vi "Initialize CAN Parameters.vi"(8 "error in (no error)":errorcluster, 11 "Diagnostics Basic Configuraiton":T24) -> (0 "error out":errorcluster, 3 "Configuration":T1={"Name"="", "Description"="", "Diagnostics Basic Configuraiton"={"Database File"=path "", "CAN Interface"=enum."CAN0", "Baud Rate"=0, "Diagnostic Protocol"=enum."GMLAN", "Transport Protocol"=enum."ISO TP - Normal Mode", "Transmit ID"=0, "Receive ID"=0, "Transmit Extension"=0, "Receive Extension"=0, "Receive UUDT ID"=0, "Enable Stream"=TRUE, "VW TP Channel ID"=0, "Security"={"DLL Path"=path "", "Security Level"=1}}, "DIDs"={"Description"="", "Frames"=[]}, "Input PIDs"={"Description"="", "Frames"=[]}, "Output PIDs"={"Description"="", "Frames"=[]}, "DPIDs"={"Description"="", "DPIDs"=[]}, "DTC"={"Description"="", "DTC descriptor"={"DTC Byte Length"=2, "Status Byte Length"=1, "Add Data Byte Length"=1, "Byte Order"=enum."Motorola"}}, "NI 986x Support"={"Enable 986x"=FALSE, "RIO Device"=0, "Bitfile"=path ""}, "Commands"={"Description"=""}, "Status"={"Description"=""}, "IO Controls"={"Description"="", "IO Control Array"=[]}, "Routines"={"Description"="", "Routine Array"=[]}, "Output Memory"={"Description"="", "Frames"=[]}, "Input Memory"={"Description"="", "Frames"=[]}} {"Input Memory"."Frames"."Signals"."Byte Order" items=["Little Endian", "Big Endian"]; "Input Memory"."Frames"."Signals"."Data Type" items=["Signed", "Unsigned", "IEEE Float"]; "Output Memory"."Frames"."Signals"."Byte Order" items=["Little Endian", "Big Endian"]; "Output Memory"."Frames"."Signals"."Data Type" items=["Signed", "Unsigned", "IEEE Float"]; "Routines"."Routine Array"."Stop Parameters"."Response"."Byte Order" items=["Little Endian", "Big Endian"]; "Routines"."Routine Array"."Stop Parameters"."Response"."Data Type" items=["Signed", "Unsigned", "IEEE Float"]; "Routines"."Routine Array"."Stop Parameters"."Cmd"."Byte Order" items=["Little Endian", "Big Endian"]; "Routines"."Routine Array"."Stop Parameters"."Cmd"."Data Type" items=["Signed", "Unsigned", "IEEE Float"]; "Routines"."Routine Array"."Request Parameters"."Response"."Byte Order" items=["Little Endian", "Big Endian"]; "Routines"."Routine Array"."Request Parameters"."Response"."Data Type" items=["Signed", "Unsigned", "IEEE Float"]; "Routines"."Routine Array"."Request Parameters"."Cmd"."Byte Order" items=["Little Endian", "Big Endian"]; "Routines"."Routine Array"."Request Parameters"."Cmd"."Data Type" items=["Signed", "Unsigned", "IEEE Float"]; "Routines"."Routine Array"."Start Parameters"."Response"."Byte Order" items=["Little Endian", "Big Endian"]; "Routines"."Routine Array"."Start Parameters"."Response"."Data Type" items=["Signed", "Unsigned", "IEEE Float"]; "Routines"."Routine Array"."Start Parameters"."Cmd"."Byte Order" items=["Little Endian", "Big Endian"]; "Routines"."Routine Array"."Start Parameters"."Cmd"."Data Type" items=["Signed", "Unsigned", "IEEE Float"]; "IO Controls"."IO Control Array"."Signals"."Response"."Byte Order" items=["Little Endian", "Big Endian"]; "IO Controls"."IO Control Array"."Signals"."Response"."Data Type" items=["Signed", "Unsigned", "IEEE Float"]; "IO Controls"."IO Control Array"."Signals"."Cmd"."Byte Order" items=["Little Endian", "Big Endian"]; "IO Controls"."IO Control Array"."Signals"."Cmd"."Data Type" items=["Signed", "Unsigned", "IEEE Float"]; "Diagnostics Basic Configuraiton"."VW TP Channel ID" format="%.0x"; "Diagnostics Basic Configuraiton"."Receive UUDT ID" format="%.0x"; "Diagnostics Basic Configuraiton"."Receive Extension" format="%.0x"; "Diagnostics Basic Configuraiton"."Transmit Extension" format="%.0x"; "Diagnostics Basic Configuraiton"."Receive ID" format="%.0x"; "Diagnostics Basic Configuraiton"."Transmit ID" format="%.0x"; "DIDs"."Frames"."Signals"."Byte Order" items=["Little Endian", "Big Endian"]; "DIDs"."Frames"."Signals"."Data Type" items=["Signed", "Unsigned", "IEEE Float"]; "Input PIDs"."Frames"."Signals"."Byte Order" items=["Little Endian", "Big Endian"]; "Input PIDs"."Frames"."Signals"."Data Type" items=["Signed", "Unsigned", "IEEE Float"]; "Output PIDs"."Frames"."Signals"."Byte Order" items=["Little Endian", "Big Endian"]; "Output PIDs"."Frames"."Signals"."Data Type" items=["Signed", "Unsigned", "IEEE Float"]})   [LabVIEW 2015, in "Diagnostics Addon System Explorer.lvlib"]
uses:
  Diagnostics Addon System Explorer.lvlib
  Shared/Base Configuration.ctl
  Shared/CAN Interface.ctl
  Shared/Diagnostic Protocols.ctl
  Shared/Exported Configuration.ctl
  Shared/CAN Configuration.ctl
  Shared/Transport Protocols.ctl
  Shared/Security.ctl
  Shared/Exported Frames Cluster.ctl
  Shared/Frame Parameters.ctl
  Shared/Signal Parameters.ctl
  Shared/Exported DPIDs Cluster.ctl
  Shared/Exported DPID Parameters.ctl
  Shared/DPID Parameters.ctl
  Shared/DPID Periodic Rate.ctl
  Shared/Exported DTC Cluster.ctl
  <vilib>/Automotive Diagnostic Command Set/Diagnostic Protocols.llb/DTC Descriptor.ctl
  Shared/Exported 986x Support.ctl
  Shared/Exported Command Cluster.ctl
  Shared/Exported Status Cluster.ctl
  Shared/Exported IO Control Cluster.ctl
  Shared/IO Control Parameters.ctl
  Shared/Input and Output Signal Parameters.ctl
  Shared/Exported Routines Cluster.ctl
  Shared/Routine Paramaters.ctl
  Shared/Diagnostics Addon Shared.lvlib
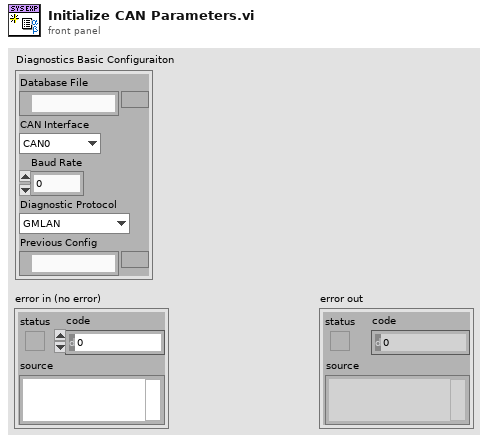
[diagram p1: front panel]
types:
  T1 = typedef "Diagnostics Addon System Explorer.lvlib/Exported Configuration.ctl" = cluster{"Name":string, "Description":string, "Diagnostics Basic Configuraiton":T2, "DIDs":T7, "Input PIDs":T7, "Output PIDs":T7, "DPIDs":T10, "DTC":T14, "NI 986x Support":T16, "Commands":T17, "Status":T18, "IO Controls":T19, "Routines":T22, "Output Memory":T7, "Input Memory":T7}
  T2 = typedef "Diagnostics Addon Shared.lvlib/CAN Configuration.ctl" = cluster{"Database File":path, "CAN Interface":T3, "Baud Rate":u32, "Diagnostic Protocol":T4, "Transport Protocol":T5, "Transmit ID":u32, "Receive ID":u32, "Transmit Extension":u8, "Receive Extension":u8, "Receive UUDT ID":u32, "Enable Stream":bool, "VW TP Channel ID":u32, "Security":T6}
  T3 = typedef "Diagnostics Addon Shared.lvlib/CAN Interface.ctl" = enum16{"CAN0", "CAN1", "CAN2", "CAN3", "CAN4", "CAN5", "CAN6", "CAN7", "CAN8", "CAN9", "CAN10", "CAN11", "CAN12", "CAN13", "CAN14", "CAN15", "CAN16", "CAN17", "CAN18", "CAN19", "CAN20", "CAN21", "CAN22", "CAN23", "CAN24", "CAN25", "CAN26", "CAN27", "CAN28", "CAN29", "CAN30", "CAN31", "CAN32", "CAN33", "CAN34", "CAN35", "CAN36", "CAN37", "CAN38", "CAN39", "CAN40", "CAN41", "CAN42", "CAN43", "CAN44", "CAN45", "CAN46", "CAN47", "CAN48", "CAN49", "CAN50", "CAN51", "CAN52", "CAN53", "CAN54", "CAN55", "CAN56", "CAN57", "CAN58", "CAN59", "CAN60", "CAN61", "CAN62", "CAN63", "CAN 256 (Virtual)", "CAN 257 (Virtual)"}
  T4 = typedef "Diagnostics Addon Shared.lvlib/Diagnostic Protocols.ctl" = enum16{"GMLAN", "KWP-2000", "UDS"}
  T5 = typedef "Diagnostics Addon Shared.lvlib/Transport Protocols.ctl" = enum16{"ISO TP - Normal Mode", "ISO TP - Mixed Mode", "VW TP 2.0", "Diagnostics on IP"}
  T6 = typedef "Diagnostics Addon Shared.lvlib/Security.ctl" = cluster{"DLL Path":path, "Security Level":u8}
  T7 = typedef "Diagnostics Addon System Explorer.lvlib/Exported Frames Cluster.ctl" = cluster{"Description":string, "Frames":T8[]}
  T8 = typedef "Diagnostics Addon Shared.lvlib/Frame Parameters.ctl" = cluster{"Name":string, "Description":string, "ID":u16, "Signals":T9[]}
  T9 = typedef "Diagnostics Addon Shared.lvlib/Signal Parameters.ctl" = cluster{"Start Bit":u8, "Length":u8, "Scaling Factor":dbl, "Scaling Offset":dbl, "Minimum":dbl, "Maximum":dbl, "Data Type":u32, "Byte Order":u32, "Default Value":dbl, "Name":string, "Units":string, "Description":string}
  T10 = typedef "Diagnostics Addon System Explorer.lvlib/Exported DPIDs Cluster.ctl" = cluster{"Description":string, "DPIDs":T11[]}
  T11 = typedef "Diagnostics Addon System Explorer.lvlib/Exported DPID Parameters.ctl" = cluster{"Name":string, "Description":string, "DPID":T12}
  T12 = typedef "Diagnostics Addon Shared.lvlib/DPID Parameters.ctl" = cluster{"DPID ID":u8, "Speed":T13, "PIDs":u16[]}
  T13 = typedef "Diagnostics Addon Shared.lvlib/DPID Periodic Rate.ctl" = enum16{"Slow", "Medium", "Fast"}
  T14 = typedef "Diagnostics Addon System Explorer.lvlib/Exported DTC Cluster.ctl" = cluster{"Description":string, "DTC descriptor":T15}
  T15 = typedef "Diagnostics Addon Shared.lvlib/DTC Descriptor.ctl" = cluster{"DTC Byte Length":i32, "Status Byte Length":i32, "Add Data Byte Length":i32, "Byte Order":enum16{"Motorola", "Intel"}}
  T16 = typedef "Diagnostics Addon System Explorer.lvlib/Exported 986x Support.ctl" = cluster{"Enable 986x":bool, "RIO Device":u16, "Bitfile":path}
  T17 = typedef "Diagnostics Addon System Explorer.lvlib/Exported Command Cluster.ctl" = cluster{"Description":string}
  T18 = typedef "Diagnostics Addon System Explorer.lvlib/Exported Status Cluster.ctl" = cluster{"Description":string}
  T19 = typedef "Diagnostics Addon System Explorer.lvlib/Exported IO Control Cluster.ctl" = cluster{"Description":string, "IO Control Array":T20[]}
  T20 = typedef "Diagnostics Addon Shared.lvlib/IO Control Parameters.ctl" = cluster{"Name":string, "Description":string, "ID":u16, "Mode":u8, "Signals":T21}
  T21 = typedef "Diagnostics Addon Shared.lvlib/Input and Output Signal Parameters.ctl" = cluster{"Cmd":T9[], "Response":T9[]}
  T22 = typedef "Diagnostics Addon System Explorer.lvlib/Exported Routines Cluster.ctl" = cluster{"Description":string, "Routine Array":T23[]}
  T23 = typedef "Diagnostics Addon Shared.lvlib/Routine Paramaters.ctl" = cluster{"Name":string, "Description":string, "ID":u16, "Start Parameters":T21, "Request Parameters":T21, "Stop Parameters":T21}
  T24 = typedef "Diagnostics Addon System Explorer.lvlib/Base Configuration.ctl" = cluster{"Database File":path, "CAN Interface":T3, "Baud Rate":u32, "Diagnostic Protocol":T4, "Previous Config":path}
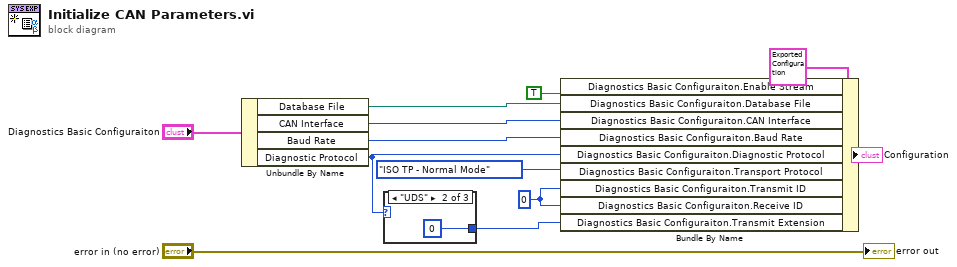
[diagram p0: block diagram]
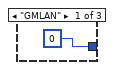
[diagram p2: hidden frame]
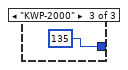
[diagram p3: hidden frame]
diagram:
  w6 = u32 0 ("Transmit ID")
  n1 = Unbundle By Name("Diagnostics Basic Configuraiton") -> ("Database File"=w11:path, "CAN Interface"=w10:T3, "Baud Rate"=w9:u32, "Diagnostic Protocol"=w8:T4)
  n2 = case shown="\"GMLAN\"" w8 {
    tunnel: [u8 0 ("Mode ID") u8 0 ("Mode ID") u8 135 ("Mode ID")] -> w4
    frame "GMLAN" {
    }
    frame "UDS" {
    }
    frame "KWP-2000" {
    }
  }
  n3 = Bundle By Name(cluster=T1 {"Name"="", "Description"="", "Diagnostics Basic Configuraiton"={"Database File"=path "", "CAN Interface"=enum."CAN0", "Baud Rate"=0, "Diagnostic Protocol"=enum."GMLAN", "Transport Protocol"=enum."ISO TP - Normal Mode", "Transmit ID"=0, "Receive ID"=0, "Transmit Extension"=0, "Receive Extension"=0, "Receive UUDT ID"=0, "Enable Stream"=TRUE, "VW TP Channel ID"=0, "Security"={"DLL Path"=path "", "Security Level"=1}}, "DIDs"={"Description"="", "Frames"=[]}, "Input PIDs"={"Description"="", "Frames"=[]}, "Output PIDs"={"Description"="", "Frames"=[]}, "DPIDs"={"Description"="", "DPIDs"=[]}, "DTC"={"Description"="", "DTC descriptor"={"DTC Byte Length"=2, "Status Byte Length"=1, "Add Data Byte Length"=1, "Byte Order"=enum."Motorola"}}, "NI 986x Support"={"Enable 986x"=FALSE, "RIO Device"=0, "Bitfile"=path ""}, "Commands"={"Description"=""}, "Status"={"Description"=""}, "IO Controls"={"Description"="", "IO Control Array"=[]}, "Routines"={"Description"="", "Routine Array"=[]}, "Output Memory"={"Description"="", "Frames"=[]}, "Input Memory"={"Description"="", "Frames"=[]}} ("Configuration"), "Diagnostics Basic Configuraiton.Enable Stream"=TRUE ("Enable Stream"), "Diagnostics Basic Configuraiton.Database File"=w11, "Diagnostics Basic Configuraiton.CAN Interface"=w10, "Diagnostics Basic Configuraiton.Baud Rate"=w9, "Diagnostics Basic Configuraiton.Diagnostic Protocol"=w8, "Diagnostics Basic Configuraiton.Transport Protocol"=Transport_Protocols."ISO TP - Normal Mode" ("Transport Protocol"), "Diagnostics Basic Configuraiton.Transmit ID"=w6, "Diagnostics Basic Configuraiton.Receive ID"=w6, "Diagnostics Basic Configuraiton.Transmit Extension"=w4) -> (→"Configuration":T1)
  "error out" <- "error in (no error)"
